vi "Quadrature Encoder dX Method (FPGA).vi"(0 "Clock":bool, 1 "Reset Enc":bool, 2 "A":bool, 3 "B":bool, 4 "Z":bool, 5 "Polarity":bool, 7 "Clock Divider":u16=1, 9 "Reset Position":i32) -> (14 "Vel/Acc Update":bool, 15 "Position (Counts)":i32, 16 "Velocity (Counts/Interval)":i32, 17 "Acceleration (Counts/Interval^2)":i32, 18 "dT (Ticks)":u32, 19 "CW Direction":bool)   [LabVIEW 2011]
doc: "Calculates 32-bit position, velocity, and acceleration based on a Quadrature encoder signal. This function resets the position upon the first Z index pulse. Subsequent Z index pulses are ignored. The velocity and acceleration values are not effected when the position is reset by the Z index pulse. The Direction input determines whether the function counts up or down based on clockwise motion.\n\nOPERATION\nUses A, B, and Z index signals to calculate position. Upon the falling edge of the Clock input, the function updates the position, velocity, acceleration, and elapsed time and latches the result. The velocity is calculated in units of Counts/Interval by subtracting the current position from the previous position. The acceleration is calculated in units of Counts/Interval^2 by subtracting the current velocity from the previous velocity.\n\nThe Clock Divider signal increases the time interval between velocity and acceleration estimates by N number of clocks to provide better resolution when the time interval between clock updates is small. Since more encoder counts are acquired during the time interval, the accuracy increases. The drawback is that the time delay also increases for the velocity and acceleration updates. The position always updates on every rising clock edge. If Clock Divider is set to 0 the Clock signal is ignored and the position, velocity, and acceleration are updated each time the function is called.\n\nThis function should be run as fast as possible to ensure that no Quadrature encoder digital edges are missed. Do not add delay timers into the loop containing this function.\n\nIf the encoder signals are noise, you may want to use the Filter Digital Lines, 3-ch (FPGA).vi function on the A, B, and Z signals before feeding them into this Quadrature encoder function.\n\nRT HOST INTERFACE\nIn your RT host application, you can divide Velocity (Counts/Interval) by the time interval dT (Ticks) to convert the velocity to units of Counts/Tick. By default, one tick is equal to 25 nanoseconds (40 MHz), so you can calculate the velocity in units of Counts per Second as follows,\n\nVelocity (Counts/s) = Velocity (Counts/Interval) / [dT (Ticks) * 25e-9 (s)]\n\nIn your RT host application, you can divide Acceleration (Counts/Interval^2) by the square of the time interval (dT (Ticks))^2 to convert the acceleration to units of Counts/Tick^2. By default, one tick is equal to 25 nanoseconds (40 MHz), so you can calculate the acceleration in units of Counts per Second^2 as follows,\n\nAcceleration (Counts/s^2) = Acceleration (Counts/Interval^2) / [(dT (Ticks))^2 * 25e-9^2 (s^2)]\n\nINPUTS\nClock- Falling edge latches the position, velocity, acceleration, and elapsed time\nReset- Sets the position to the Reset Position value\nA- Quadrature encoder A phase signal\nB- Quadrature encoder B phase signal\nZ- Quadrature encoder Z index signal\nPolarity- When FALSE, counterclockwise motion causes the Position (Counts) output to increment\nClock Divider- Causes the velocity and acceleration values to update every N clocks\nReset Position- The position will be set to this value when the first Z index pulse occurs or the Reset input is asserted\nVel/Acc Update- Boolean signal that changes state when the velocity and acceleration outputs are updated. Used for synchronization with other loops.\nCW Direction- If the Polarity input is FALSE, this signal is TRUE when clockwise motion is detected\n\n\nOUTPUTS\nPosition (Counts)- The position count value, updated continuously\nVelocity (Counts/Interval)- The amount the position has changed between the last two updates\nAcceleration (Counts/Interval^2)- The amount the velocity has changed between the last two updates\ndT (Ticks)- The time interval between velocity and acceleration updates, express in FPGA clock ticks\n\nNOTES\nBy allowing more time between updates you obtain more averaging on the velocity and acceleration values and therefore smoother results. A larger time interval results in less noise on the velocity and acceleration calculations. Also, using an encoder with more counts per revolution results in better accuracy and smoother results on the velocity and acceleration calculations.\n\nSaturation Subtract functions are used to saturate the signed velocity and acceleration values in the case of integer overflow. \n\nA normal Subtract function is used on the elapsed time counter. Because unsigned integers are used, the dT (Ticks) value is correct even when the Tick Count value rolls over."
uses:
  <vilib>/Platform/TimedLoop/XDataNode/timing_clust.ctl
  <vilib>/Platform/TimedLoop/XDataNode/nitl_modes.ctl
  <vilib>/Platform/TimedLoop/XDataNode/wakeup.ctl
  <vilib>/Platform/TimedLoop/XDataNode/XDataNode.xnode
  <vilib>/rvi/Arithmetic/AddSubMult/XNode/nirviSatArithmetic.xnode
  <vilib>/Platform/TimedLoop/XDataNode/XDNodeRunTimeDep.lvlib
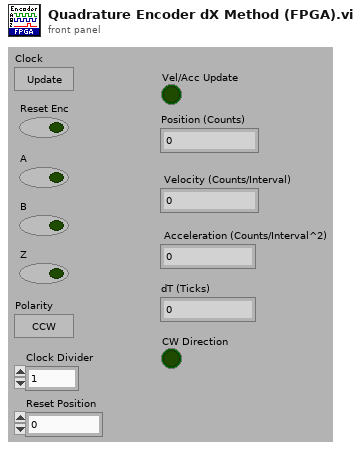
[diagram p1: front panel]
types:
  T1 = typedef "XDNodeRunTimeDep.lvlib/timing_clust.ctl" = cluster{"Expected End [f-1]":u64, "Actual End [f-1]":u64, "Finished Late? [f-1]":bool, "Expected End [i-1]":u64, "Actual End [i-1]":u64, "Finished Late? [i-1]":bool, "Expected Start [i]":u64, "Actual Start [i]":u64, "Expected Start [f]":u64, "Actual Start [f]":u64, "Source Name":string, "Structure Name":string, "Period":i64, "Deadline":i64, "Offset":i64, "Start":i64, "Priority":i32, "Timeout":i32, "Mode":T2, "Wakeup Reason":T3, "Error":errorcluster, "Source Type":string, "Secondary Source Type":string, "Global End Time":u64, "Global Start Time":u64, "Frame Duration":u64, "Iteration Duration":u64, "Assigned CPU":i32, "I/O Scan Engine Mode":u32}
  T2 = typedef "XDNodeRunTimeDep.lvlib/nitl_modes.ctl" = enum32{"No Change", "Process missed periods, maintain original phase", "Discard missed periods, maintain original phase", "Process missed periods, ignore original phase", "Discard missed periods, ignore original phase"}
  T3 = typedef "XDNodeRunTimeDep.lvlib/wakeup.ctl" = enum32{"Normal", "Aborted", "Asynchronous wakeup", "Timing source error", "Timed loop error", "Timeout"}
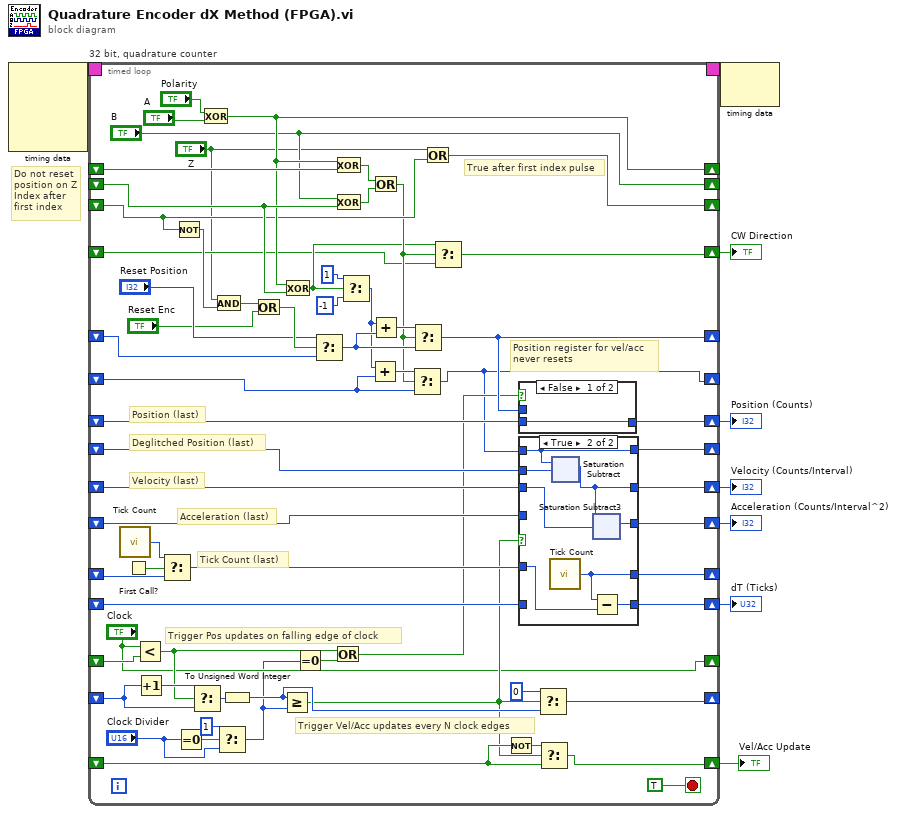
[diagram p0: block diagram]
diagram:
  # "Do not reset position on Z Index after first index"
  n1 = node-c288() -> (w4:T1)  [unwired: 4 in]
  n2 = timed-loop "32 bit, quadrature counter" {
    shift-right: [w62] -> _
    shift-left: _ -> [w69]
    shift-right: [w46] -> _
    shift-left: _ -> [w57]
    shift-right: ["B"] -> _
    shift-left: _ -> [w66]
    shift-right: [w51] -> _
    shift-left: _ -> [w64]
    shift-right: [w54] -> w7
    shift-left: _ -> [w63]
    shift-right: [w53] -> w6
    shift-left: _ -> [w61]
    shift-right: [w60] -> _
    shift-left: _ -> [w59]
    shift-right: [w31] -> _
    shift-left: _ -> [w30]
    shift-right: [w56] -> w5
    shift-left: _ -> [w55]
    shift-right: [w52] -> _
    shift-left: _ -> [w49]
    shift-right: [w44] -> w8
    shift-left: _ -> [w45]
    shift-right: ["Clock"] -> _
    shift-left: _ -> [w47]
    shift-right: [w29] -> _
    shift-left: _ -> [w41]
    timing: w4 -> [_]
    timing-out: [_] -> w3
    shift-right: [w27] -> w2
    shift-left: _ -> [w26]
    shift-right: [w21] -> w1
    shift-left: _ -> [w20]
    stop <- TRUE ("stop") stop-if-true
    # "Trigger Vel/Acc updates every N clock edges"
    # "Trigger Pos updates on falling edge of clock"
    # "Position (last)"
    # "Tick Count (last)"
    # "Position register for vel/acc\nnever resets"
    # "True after first index pulse"
    # "Acceleration (last)"
    # "Velocity (last)"
    # "Deglitched Position (last)"
    n3 = call "Tick Count"() -> ("Tick Count(Ticks)"=w14:u32)
    n4 = First Call?() -> (First Call?: T/F=w50:bool)
    n5 = Less?(x="Clock", y=w47) -> (x < y?=w40:bool)
    n6 = Increment(x=w41) -> (x+1=w43:u16)
    n7 = Select(t=w14, s=w50, f=w49) -> (s? t:f=w48:u32)
    n8 = Not(x=w59) -> (.not. x?=w58:bool)
    n9 = Equal To 0?(x="Clock Divider") -> (x = 0?=w12:bool)
    n10 = Select(t=w43, s=w40, f=w41) -> (s? t:f=w42:u16)
    n11 = Exclusive Or(1:"A", 2:"Polarity") -> (0:w62:bool)
    n12 = And(x="Z", y=w58) -> (x .and. y?=w35:bool)
    n13 = Select(t=u16 1, s=w12, f="Clock Divider") -> (s? t:f=w9:u16)
    n14 = To Unsigned Word Integer(number=w42) -> (unsigned 16bit integer=w39:u16)
    n15 = Or(x=w35, y="Reset Enc") -> (x .or. y?=w34:bool)
    n16 = Greater Or Equal?(x=w39, y=w9) -> (x >= y?=w25:bool)
    n17 = Exclusive Or(1:w66, 2:w62) -> (0:w22:bool)
    n18 = Equal To 0?(x=w9) -> (x = 0?=w36:bool)
    n19 = Select(t="Reset Position", s=w34, f=w57) -> (s? t:f=w72:i32)
    n20 = Or(x=w40, y=w36) -> (x .or. y?=w37:bool)
    n21 = Exclusive Or(1:w69, 2:w62) -> (0:w67:bool)
    n22 = Exclusive Or(1:w66, 2:"B") -> (0:w68:bool)
    n23 = Select(t=1 ("32 bit"), s=w22, f=-1 ("32 bit")) -> (s? t:f=w32:i32)
    n24 = Add(x=w32, y=w30) -> (x+y=w33:i32)
    n25 = Or(x=w67, y=w68) -> (x .or. y?=w23:bool)
    n26 = Add(x=w32, y=w72) -> (x+y=w73:i32)
    n27 = Select(t=w33, s=w23, f=w30) -> (s? t:f=w31:i32)
    n28 = Select(t=w73, s=w23, f=w72) -> (s? t:f=w46:i32)
    n29 = Or(x="Z", y=w59) -> (x .or. y?=w60:bool)
    n30 = Select(t=w22, s=w23, f=w20) -> (s? t:f=w21:bool)
    n31 = Not(x=w26) -> (.not. x?=w28:bool)
    n32 = case shown="False" w37 {
      tunnel: w46 -> [_ w75]
      tunnel: w45 -> [w74 _]
      tunnel: [w74 w75] -> w44
      frame False {
      }
      frame True {
      }
    }
    n33 = case shown="True" w25 {
      tunnel: w31 -> [_ w88]
      tunnel: [w80 w88] -> w51
      tunnel: w64 -> [w80 w87]
      tunnel: [w79 w86] -> w54
      tunnel: w63 -> [w79 w85]
      tunnel: [w78 w84] -> w53
      tunnel: w61 -> [w78 _]
      tunnel: [w77 w83] -> w56
      tunnel: w55 -> [w77 _]
      tunnel: [w76 w82] -> w52
      tunnel: w48 -> [w76 w81]
      frame False {
      }
      frame True {
        n34 = call "Tick Count"() -> ("Tick Count(Ticks)"=w82:u32)
        n35 = xnode ("Saturation Subtract")("x"=w88, "y"=w87) -> ("x-y"=w86:i32)
        n36 = Subtract(x=w82, y=w81) -> (x-y=w83:u32)
        n37 = xnode ("Saturation Subtract3")("x"=w86, "y"=w85) -> ("x-y"=w84:i32)
      }
    }
    n38 = Select(t=u16 0, s=w25, f=w39) -> (s? t:f=w29:u16)
    n39 = Select(t=w28, s=w25, f=w26) -> (s? t:f=w27:bool)
  }
  "Position (Counts)" <- w8
  "Velocity (Counts/Interval)" <- w7
  "Acceleration (Counts/Interval^2)" <- w6
  "dT (Ticks)" <- w5
  "Vel/Acc Update" <- w2
  "CW Direction" <- w1
  n40 = node-c288(w3) -> ()  [unwired: 1 out]
